vi "__testPrintStack.vi"() -> ()   [LabVIEW 2011]
panel:
  out "数组":string[](array[string])
  out "lua_type":i32(ring) items=["LUA_TNONE"=-1, "LUA_TNIL"=0, "LUA_TBOOLEAN"=1, "LUA_TLIGHTUSERDATA"=2, "LUA_TNUMBER "=3, "LUA_TSTRING"=4, "LUA_TTABLE"=5, "LUA_TFUNCTION"=6, "LUA_TUSERDATA"=7, "LUA_TTHREAD"=8, "LUA_NUMTAGS "=9]
  in  "lua_State *L":u64
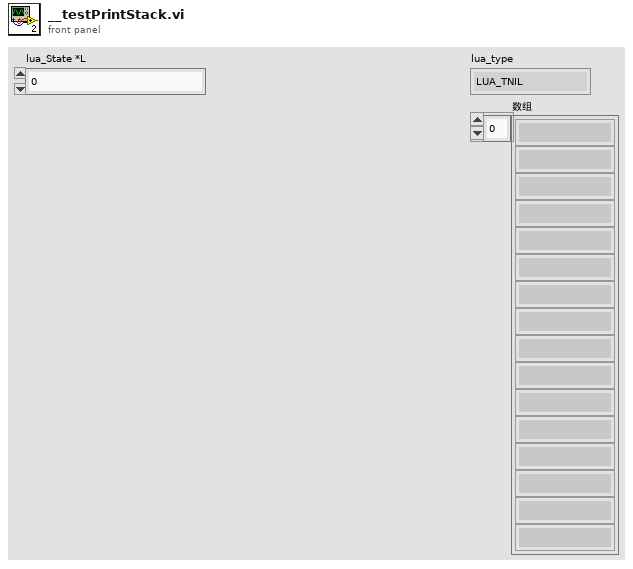
[diagram p1: front panel]
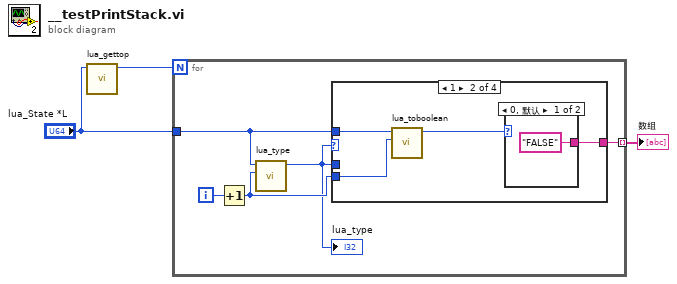
[diagram p0: block diagram]
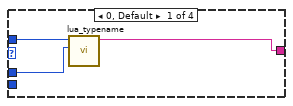
[diagram p2: hidden frame]
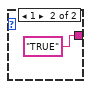
[diagram p3: hidden frame]
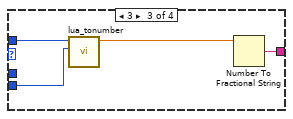
[diagram p4: hidden frame]
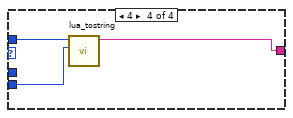
[diagram p5: hidden frame]
diagram:
  n1 = call "lua_gettop.vi"("lua_State *L"="lua_State *L") -> ("lua_gettop"=w3:i32)  [unwired: 9 in, 1 out]
  n2 = for {
    N: w3 -> [_]
    tunnel: "lua_State *L" -> [w7]
    tunnel: [w5] -> w1 mode=indexing
    i -> [w8]
    n3 = Increment(x=w8) -> (x+1=w6:i32)
    n4 = call "lua_type.vi"("int index"=w6, "lua_State *L"=w7) -> ("lua_type"=w4:i32)  [unwired: 8 in, 1 out]
    "lua_type" <- w4
    n5 = case shown="1" w4 {
      tunnel: w7 -> [w10 w15 w21 w24]
      tunnel: w6 -> [_ w14 w20 w23]
      tunnel: [w11 w12 w18 w22] -> w5
      tunnel: w4 -> [w9 _ _ _]
      frame 0, Default {
        n6 = call "lua_typename.vi"("int tp"=w9, "lua_State *L"=w10) -> ("lua_typename"=w11:string)  [unwired: 8 in, 1 out]
      }
      frame 1 {
        n7 = call "lua_toboolean.vi"("index"=w14, "lua_State *L"=w15) -> ("lua_toboolean"=w13:i32)  [unwired: 8 in, 1 out]
        n8 = case shown="0, 默认" w13 {
          tunnel: ["FALSE" "TRUE"] -> w12
          frame 0, Default {
          }
          frame 1 {
          }
        }
      }
      frame 3 {
        n9 = call "lua_tonumber.vi"("index"=w20, "lua_State *L"=w21) -> ("lua_Number"=w19:dbl)  [unwired: 8 in, 1 out]
        n10 = Number To Fractional String(number=w19) -> (F-format string=w18:string)  [unwired: 3 in]
      }
      frame 4 {
        n11 = call "lua_tostring.vi"("index"=w23, "lua_State *L"=w24) -> ("constant string"=w22:string)  [unwired: 8 in, 1 out]
      }
    }
  }
  "数组" <- w1
